vi "Lv_DEMO.vi"() -> ()   [LabVIEW 2015]
uses:
  C:/Users/Way/source/repos/MACOs.JY.ActorFramework/examples/Lv_DEMO/TestService.dll
  TestService.dll
  C:/Users/Way/source/repos/MACOs.JY.ActorFramework/examples/net472_DEMO/bin/Debug/MACOs.JY.ActorFramework.Core.dll
  net472_DEMO/bin/Debug/MACOs.JY.ActorFramework.Core.dll
  C:/Users/Way/source/repos/MACOs.JY.ActorFramework/examples/net472_DEMO/bin/Debug/MACOs.JY.ActorFramework.Clients.dll
  net472_DEMO/bin/Debug/MACOs.JY.ActorFramework.Clients.dll
  C:/Users/Way/source/repos/MACOs.JY.ActorFramework/examples/Lv_DEMO/MACOs.JY.ActorFramework.Implement.NetMQ.dll
  MACOs.JY.ActorFramework.Implement.NetMQ.dll
panel:
  out "error out":errorcluster
  in  "stop":bool
  in  "OK Button":bool
  out "Output String":string
  in  "Input String":string
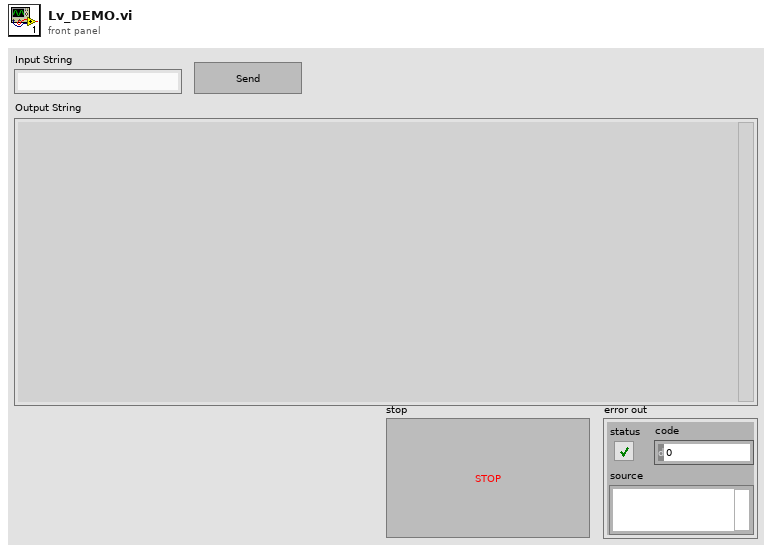
[diagram p1: front panel]
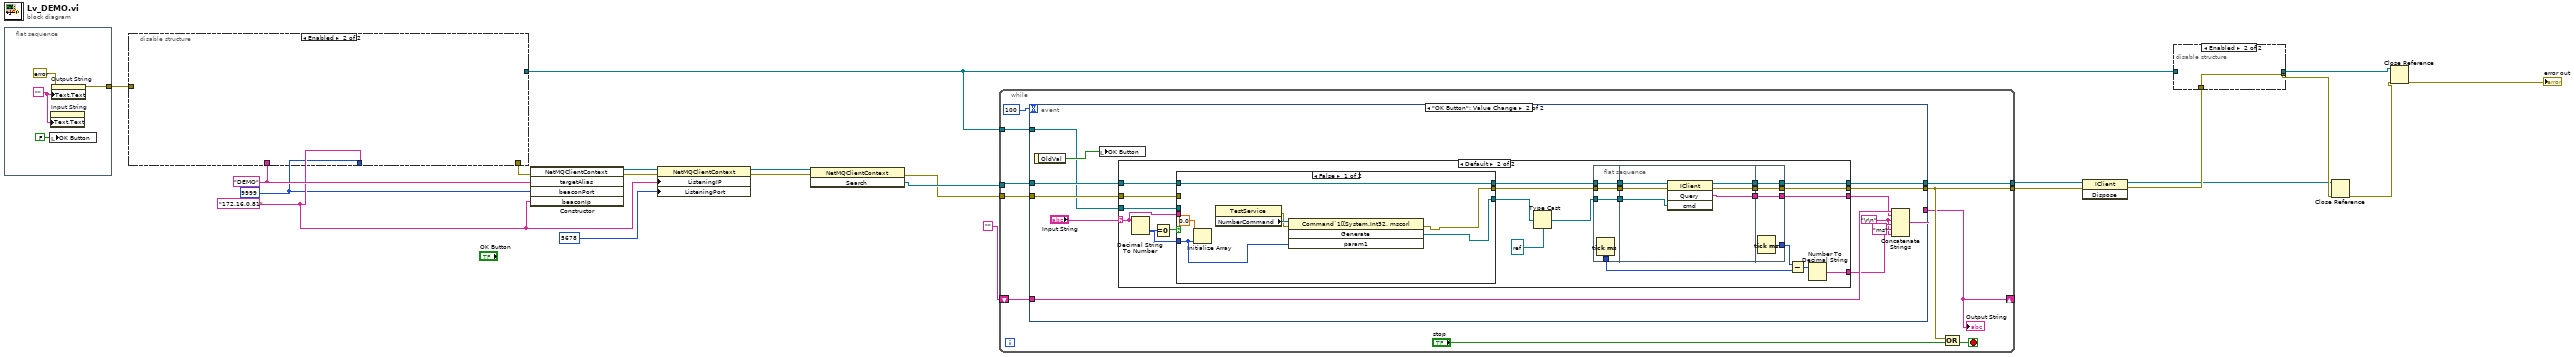
[diagram p0: block diagram]
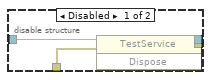
[diagram p2: hidden frame]
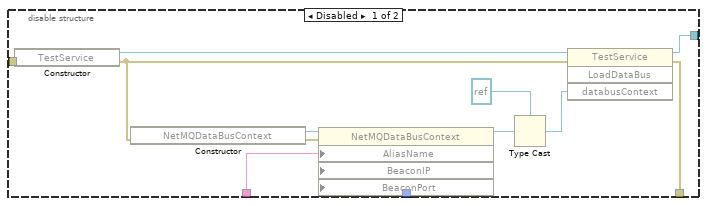
[diagram p3: hidden frame]
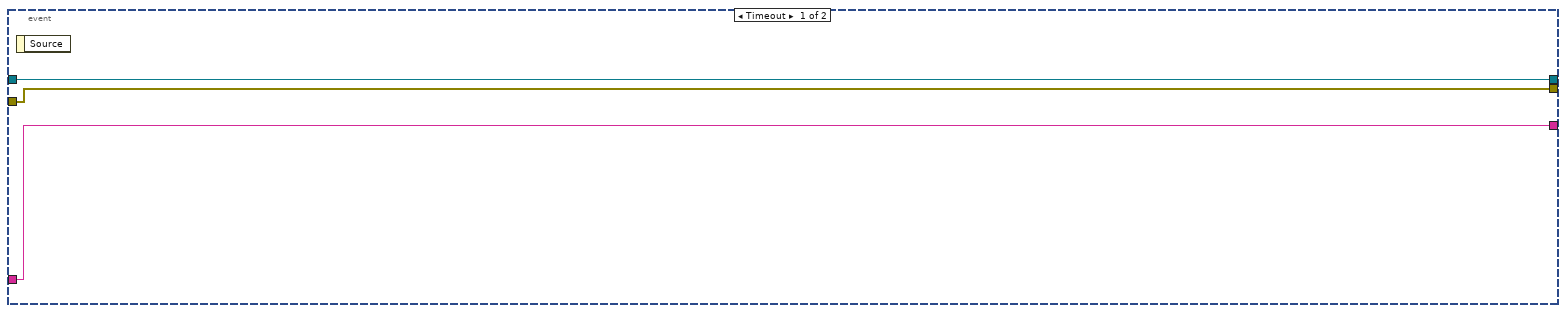
[diagram p4: hidden frame]
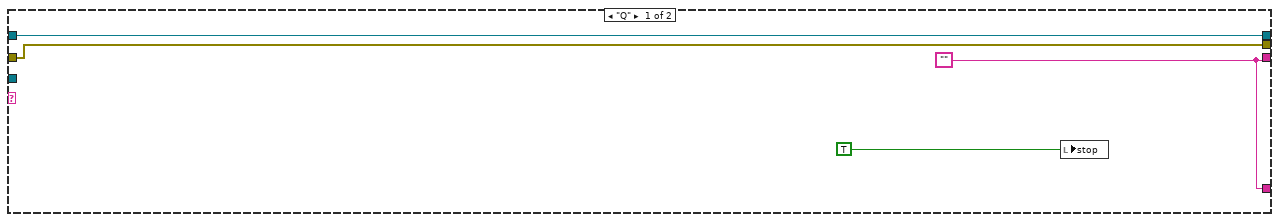
[diagram p5: hidden frame]
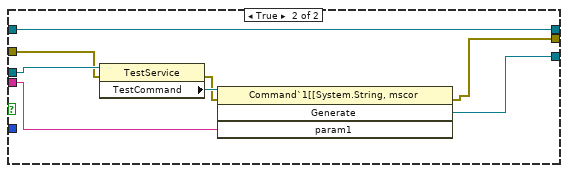
[diagram p6: hidden frame]
diagram:
  w2 = "172.16.0.81" ("alias")
  w11 = "DEMO" ("alias")
  w1 = 9999 ("port")
  n1 = flat-sequence {
    tunnel: [w26] -> w14
    frame #0 {
      w25 = ""
      n2 = local write "OK Button"(FALSE ("OK Button")) -> ()
      n3 = property on="Input String" class="Str"("Text.Text"=w25) -> ()  [unwired: 2 in, 2 out]
      n4 = property on="Output String" class="Str"(error in=errorcluster {"status"=FALSE, "code"=0, "source"=""} ("error in (no error)"), "Text.Text"=w25) -> (error out=w26:errorcluster)  [unwired: 1 in, 1 out]
    }
  }
  n5 = disable-structure shown="Enabled" {
    disable-tunnel: w14 -> [w39 _]
    disable-tunnel: [w37 _] -> w12
    disable-tunnel: w11 -> [w30 _]
    disable-tunnel: [w29 _] -> w10
    disable-tunnel: w2 -> [w28 _]
    disable-tunnel: w1 -> [w27 _]
    frame Disabled {
      n6 = constructor class="TestService"(error in=w39) -> (reference out=w38:refnum<k24>, error out=w36:errorcluster)  [unwired: 2 in, 1 out]
      n7 = constructor class="NetMQDataBusContext"(error in=w36) -> (reference out=w35:refnum<k24>, error out=w34:errorcluster)  [unwired: 2 in, 1 out]
      n8 = property class="NetMQDataBusContext"(reference=w35, error in=w34, "AliasName"=w30, "BeaconIP"=w28, "BeaconPort"=w27) -> (reference out=w33:refnum<k24>)  [unwired: 1 out]
      n9 = Type Cast(type=refnum<k24> refnum ("databusContext"), x=w33) -> (*(type *) &x=w32:refnum<k24>)
      n10 = invoke class="TestService" method="LoadDataBus"(reference=w38, error in=w36, "databusContext"=w32) -> (reference out=w37:refnum<k24>, error out=w29:errorcluster)  [unwired: 1 in, 2 out]
    }
    frame Enabled {
    }
  }
  n11 = constructor class="NetMQClientContext"(error in=w10, "targetAlias"=w11, "beaconPort"=w1, "beaconIp"=w2) -> (reference out=w7:refnum<k24>, error out=w6:errorcluster)  [unwired: 2 in, 4 out]
  n12 = property class="NetMQClientContext"(reference=w7, error in=w6, "ListeningIP"=w2, "ListeningPort"=5678) -> (reference out=w4:refnum<k24>, error out=w5:errorcluster)
  n13 = invoke class="NetMQClientContext" method="Search"(reference=w4, error in=w5) -> (error out=w8:errorcluster, "Search"=w9:refnum<k24>)  [unwired: 1 in, 1 out]
  n14 = while {
    tunnel: w9 -> [w48]
    tunnel: [w44] -> w22
    tunnel: [w47] -> w21
    tunnel: w8 -> [w43]
    shift-right: [w41] -> _
    shift-left: "" -> [w42]
    tunnel: w12 -> [w40]
    stop <- w45 stop-if-true
    n15 = event shown="[1] \"OK Button\": Value Change" {
      selector: _ -> [_ _]
      dyn-events: _ -> [_ _]
      timeout: 100 -> [_ _]
      tunnel: w48 -> [w52 w65]
      tunnel: [w50 w64] -> w44
      tunnel: [w52 w63] -> w47
      tunnel: w43 -> [w50 w62]
      tunnel: w42 -> [w51 w61]
      tunnel: [w51 w59] -> w41
      tunnel: w40 -> [_ w53]
      event Timeout {
        n16 = event-data() -> ()  [unwired: 1 in, 1 out]
      }
      event "OK Button": Value Change {
        w54 = "\r\n"
        n17 = event-data() -> ("OldVal"=w57:bool)  [unwired: 1 in]
        n18 = local write "OK Button"(w57) -> ()
        n19 = case shown="Default" "Input String" {
          selector: "Input String" -> [_ w85]
          tunnel: w65 -> [w67 w93]
          tunnel: [w69 w90] -> w64
          tunnel: [w67 w89] -> w63
          tunnel: w62 -> [w69 w88]
          tunnel: [w66 w87] -> w60
          tunnel: [w66 w77] -> w56
          tunnel: w53 -> [_ w73]
          frame "Q" {
            w66 = ""
            n20 = local write "stop"(TRUE ("stop")) -> ()
          }
          frame Default {
            n21 = Decimal String To Number(string=w85) -> (number=w84:i32)  [unwired: 2 in, 1 out]
            n22 = Equal To 0?(x=w84) -> (x = 0?=w86:bool)
            n23 = case shown="False" w86 {
              tunnel: w93 -> [w113 w122]
              tunnel: [w110 w116] -> w92
              tunnel: [w113 w122] -> w91
              tunnel: w88 -> [_ w120]
              tunnel: w85 -> [_ w118]
              tunnel: w84 -> [w108 _]
              tunnel: [w109 w115] -> w72
              tunnel: w73 -> [_ w121]
              frame False {
                n24 = Initialize Array(0.0, w108) -> ()  [unwired: 1 out]
                n25 = property class="TestService"() -> (error out=w111:errorcluster, "NumberCommand"=w112:refnum<k24>)  [unwired: 2 in, 1 out]
                n26 = invoke class="Command`1[[System.Int32, mscorl" method="Generate"(reference=w112, error in=w111, "param1"=w108) -> (error out=w110:errorcluster, "Generate"=w109:refnum<k24>)  [unwired: 1 in, 2 out]
              }
              frame True {
                n27 = property class="TestService"(reference=w121, error in=w120) -> (error out=w117:errorcluster, "TestCommand"=w119:refnum<k24>)  [unwired: 1 out]
                n28 = invoke class="Command`1[[System.String, mscor" method="Generate"(reference=w119, error in=w117, "param1"=w118) -> (error out=w116:errorcluster, "Generate"=w115:refnum<k24>)  [unwired: 1 in, 2 out]
              }
            }
            n29 = Type Cast(type=refnum<k24> refnum ("cmd"), x=w72) -> (*(type *) &x=w71:refnum<k24>)
            n30 = flat-sequence {
              tunnel: w91 -> [w96]
              tunnel: w92 -> [w97]
              tunnel: [w97] -> w82
              tunnel: [w96] -> w81
              tunnel: [w95] -> w79
              tunnel: [w94] -> w76
              tunnel: w71 -> [w94]
              tunnel: [w101] -> w83
              tunnel: w82 -> [w99]
              tunnel: w81 -> [w103]
              tunnel: w76 -> [w98]
              tunnel: [w102] -> w75
              tunnel: [w100] -> w74
              tunnel: [w105] -> w87
              tunnel: [w106] -> w89
              tunnel: [w107] -> w90
              tunnel: w83 -> [w107]
              tunnel: [w104] -> w80
              tunnel: w75 -> [w105]
              tunnel: w74 -> [w106]
              frame #0 {
                n31 = Tick Count (ms)() -> (millisecond timer value=w95:u32)
              }
              frame #1 {
                n32 = invoke class="IClient" method="Query"(reference=w103, error in=w99, "cmd"=w98) -> (reference out=w100:refnum<k24>, error out=w101:errorcluster, "Query"=w102:string)  [unwired: 1 in, 1 out]
              }
              frame #2 {
                n33 = Tick Count (ms)() -> (millisecond timer value=w104:u32)
              }
            }
            n34 = Subtract(x=w80, y=w79) -> (x-y=w78:u32)
            n35 = Number To Decimal String(number=w78) -> (decimal integer string=w77:string)  [unwired: 1 in]
          }
        }
        n36 = Concatenate Strings(w61, w60, w54, w56, "ms" ("string"), w54) -> (w59:string)
      }
    }
    "Output String" <- w41
    n37 = Compound Arithmetic op=OR(w44, "stop") -> (w45:bool)
  }
  n38 = invoke class="IClient" method="Dispose"(reference=w21, error in=w22) -> (reference out=w15:refnum<k24>, error out=w19:errorcluster)  [unwired: 1 in, 1 out]
  n39 = disable-structure shown="Enabled" {
    disable-tunnel: w19 -> [w126 w127]
    disable-tunnel: [w125 w127] -> w18
    disable-tunnel: [w124 _] -> w16
    disable-tunnel: w12 -> [w123 _]
    frame Disabled {
      n40 = invoke class="TestService" method="Dispose"(reference=w123, error in=w126) -> (reference out=w124:refnum<k24>, error out=w125:errorcluster)  [unwired: 1 in, 1 out]
    }
    frame Enabled {
    }
  }
  n41 = Close Reference(reference=w15, error in (no error)=w18) -> (error out=w20:errorcluster)
  n42 = Close Reference(reference=w16, error in (no error)=w20) -> (error out=→"error out":errorcluster)
